vi "Host Approach Retraction2.vi"() -> ()   [LabVIEW 2012]
uses:
  <vilib>/FPGAPlugInAG/PCI-7831R/niLvFpga_Open_PCI-7831R.vi
  <vilib>/rvi/interface/common/dynamic/niFpgaDynamicAddResources.vi
  <vilib>/Utility/error.llb/Error Cluster From Error Code.vi
  <vilib>/rvi/errors/niLvFpgaAdjustHostInterfaceError.vi
  <vilib>/FPGAPlugInAG/Dynamic/niLvFpga_Close_Dynamic.vi
  <vilib>/FPGAPlugInAG/Dynamic/niLvFpga_Run_Dynamic.vi
  <vilib>/rvi/interface/nirviOpenFPGA/nirviOpenFPGA.xnode
  SB130-XPS/Documents/FPGA-project-apporach-retraction/FPGA Bitfiles/Apporach-Retract_FPGATarget2_FPGATargetApproa_XKCjVnL+Gdg.lvbitx
  FPGA Target Approach Retraction2.vi
  <vilib>/rvi/interface/nirviReadWriteControl/nirviReadWriteControl.xnode
  <vilib>/rvi/interface/nirviCloseFPGA/nirviCloseFPGA.xnode
  <vilib>/rvi/interface/nirviMethod/nirviMethod.xnode
  <vilib>/rvi/interface/Simulation/niFpgaSimulationCallBeginRW.vi
  NiFpgaLv.dll
  <vilib>/FPGAPlugInAG/Dynamic/niLvFpga_StartFifo_Dynamic.vi
  <vilib>/rvi/errors/niLvFpgaMergeErrorWithErrorCode.vi
  <vilib>/FPGAPlugInAG/Dynamic/niLvFpga_StopFifo_Dynamic.vi
  <vilib>/FPGAPlugInAG/Dynamic/niLvFpga_ReadFifo_Dynamic.vi
panel:
  in  "Data Acquisition Rate":i32=8000
  out "HV/10":i32[](graph)=[6085, 6084, 6081, 6089, 6083, 6081, 6089, 6086, 6085, 6082, 6090, 6078, 6083, 6081, 6081, 6075, 6082, 6084, 6094, 6094, 6097, 6092, 6083, 6084, 6094, 6085, 6094, 6088, 6085, 6088, 6096, 6079, 6078, 6091, 6099, 6071, 6086, 6086, 6087, 6089, 6086, 6098, 6098, 6101, 6089, 6094, 6083, 6073, 6082, 6086, 6085, 6090, 6084, 6082, 6084, 6084, 6078, 6085, 6094, 6082, 6089, 6088, 6086, 6080, 6087, 6083, 6084, 6082, 6087, 6085, 6079, 6086, 6093, 6085, 6077, 6092, 6081, 6078, 6075, 6072, 6079, 6085, 6084, 6078, 6073, 6090, 6082, 6078, 6088, 6090, 6082, 6098, 6082, 6088, 6079, 6084, 6085, 6084, 6083, 6086]
  out "Tuning Fork":i32[](graph)=[27033, 27029, 27028, 27032, 27032, 27030, 27031, 27032, 27030, 27031, 27034, 27037, 27037, 27035, 27036, 27035, 27030, 27033, 27036, 27034, 27037, 27033, 27030, 27030, 27031, 27025, 27032, 27032, 27032, 27034, 27032, 27032, 27032, 27033, 27029, 27032, 27036, 27032, 27030, 27033, 27031, 27033, 27037, 27036, 27034, 27032, 27032, 27034, 27033, 27032, 27032, 27030, 27029, 27029, 27033, 27033, 27029, 27029, 27033, 27036, 27036, 27033, 27033, 27034, 27033, 27033, 27035, 27033, 27032, 27033, 27032, 27032, 27034, 27036, 27034, 27032, 27035, 27036, 27032, 27036, 27034, 27032, 27032, 27036, 27036, 27033, 27038, 27036, 27033, 27034, 27035, 27032, 27030, 27034, 27039, 27037, 27029, 27033, 27033, 27033]
  in  "Number of Elements":i32=100
  out "Counter Indicator":i32(graph)=-27
  out "Z Indicator":dbl(graph)=30.0
  out "FPGA Output Voltage":dbl(graph)=-0.00824931263923645
  in  "MCL Counter":i64=100
  in  "MCL Divisions":i32=200
  out "MCL Range Indicator":bool=TRUE
  out "Host Counter Indicator":i64=100
  out "Digital Steps per Region":i32=327
  out "Host Counter Output":i32=-27
  in  "Z Position MCL Fine":i32=6000
  out "Host Z Position Indicator":i32=6000
  out "Z Position Range Indicator":bool=TRUE
  out "Z Fine Steps per Region":dbl=0.0049897001602197295
  out "Host Z Output":fxp<+/-,40,30>=29.9384765625
  in  "Manual Approach Start":bool
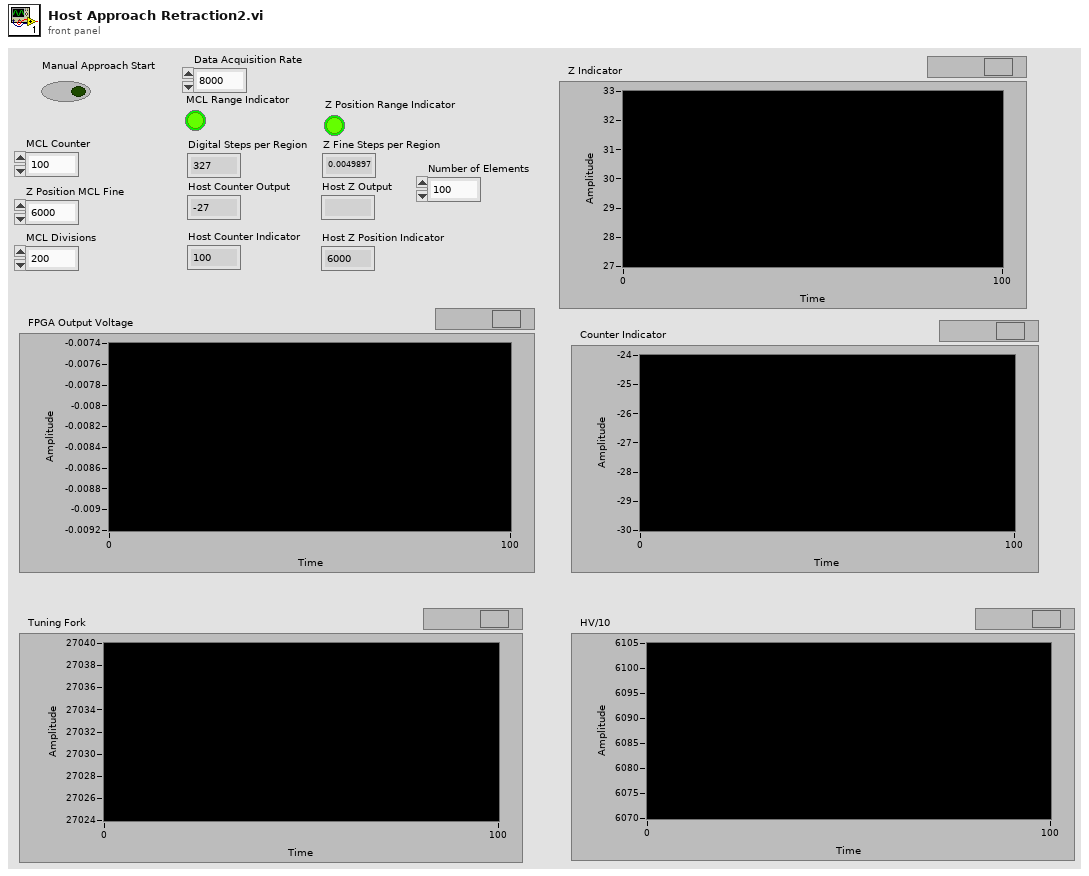
[diagram p1: front panel]
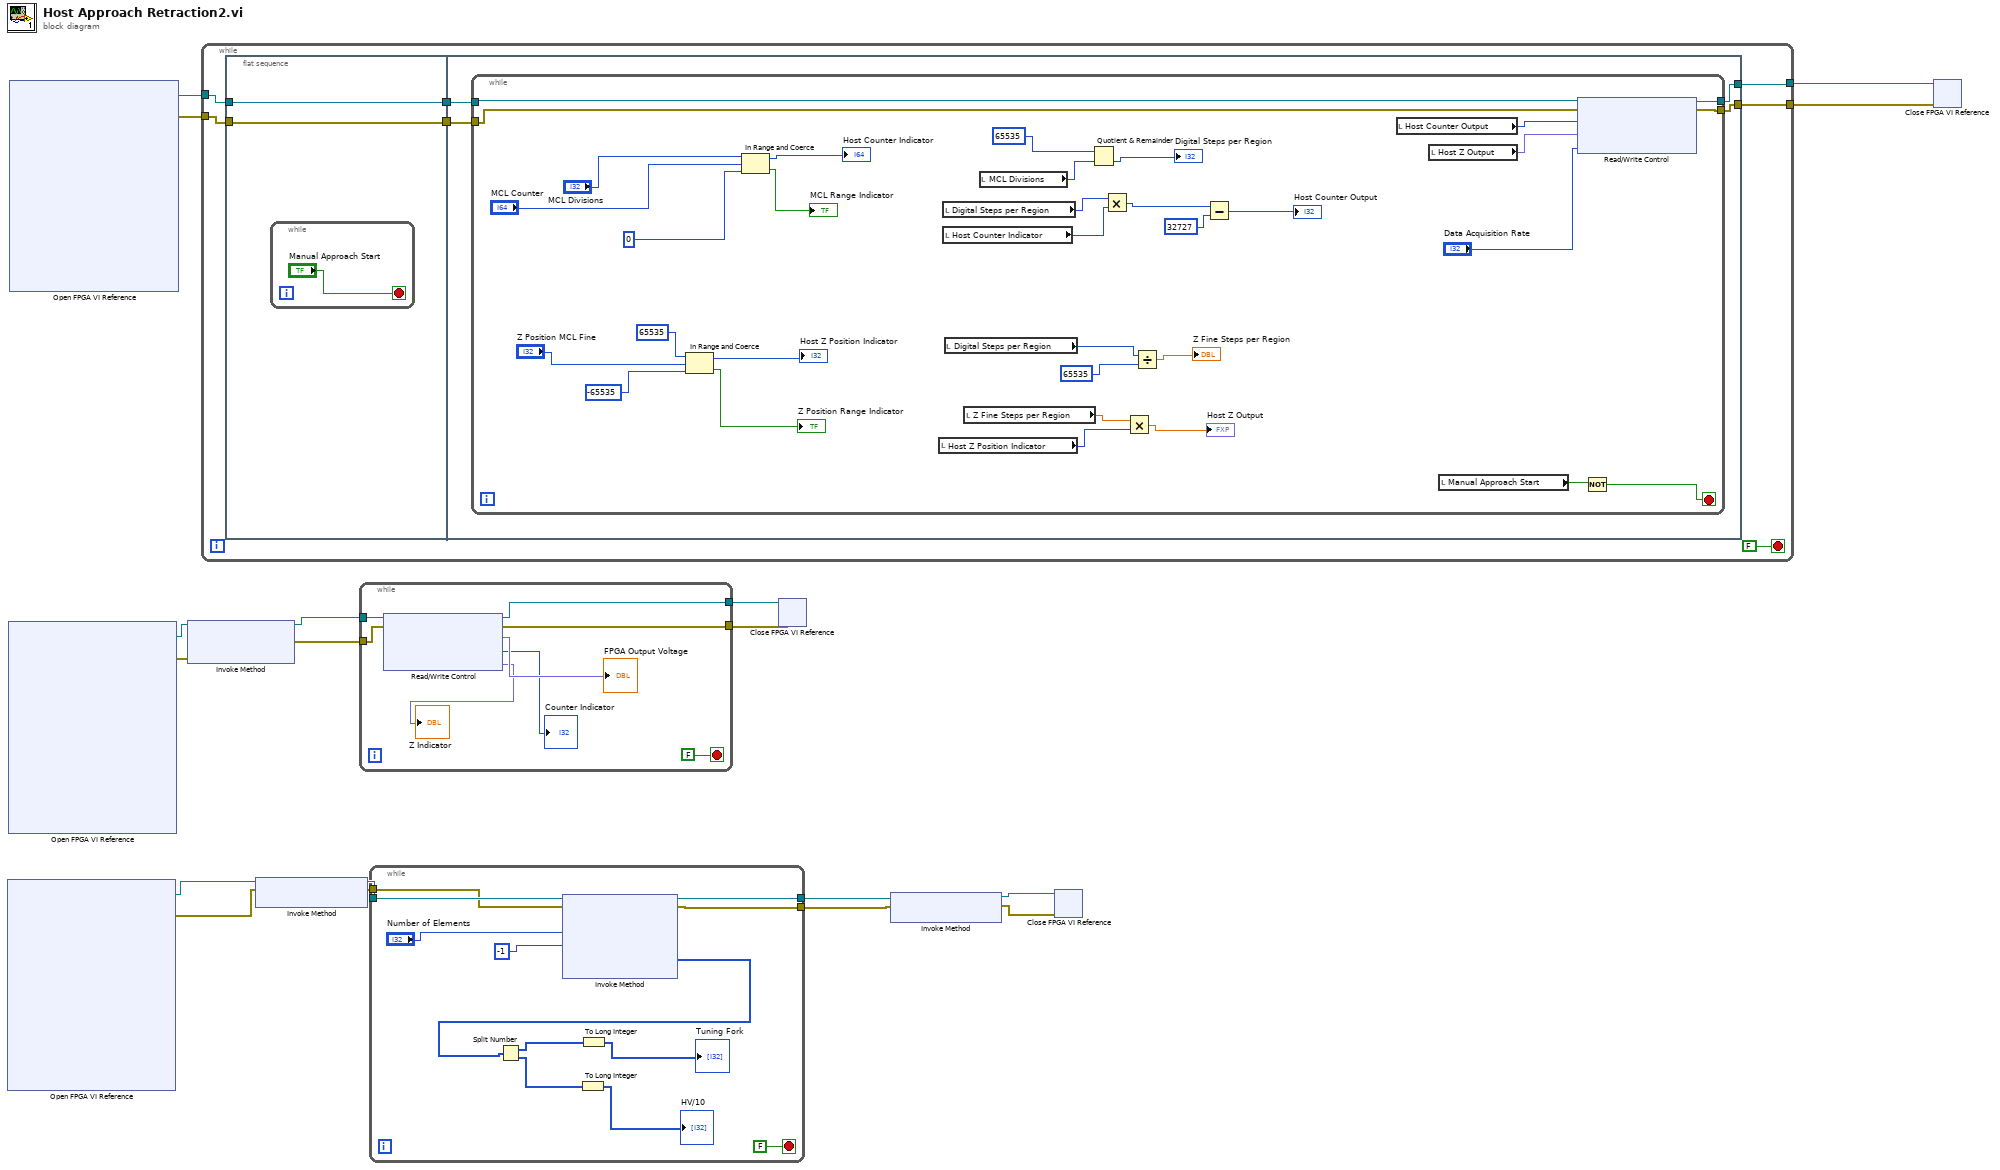
[diagram p0: block diagram]
diagram:
  n1 = xnode "Open FPGA VI Reference"() -> ("FPGA VI Reference Out"=w8:refnum<k20>, "error out"=w7:errorcluster)  [unwired: 2 in]
  n2 = xnode "Open FPGA VI Reference"() -> ("FPGA VI Reference Out"=w10:refnum<k20>, "error out"=w9:errorcluster)  [unwired: 2 in]
  n3 = xnode "Open FPGA VI Reference"() -> ("FPGA VI Reference Out"=w16:refnum<k20>, "error out"=w15:errorcluster)  [unwired: 2 in]
  n4 = xnode "Invoke Method"("FPGA VI Reference In"=w10, "error in"=w9) -> ("FPGA VI Reference Out"=w12:refnum<k20>, "error out"=w11:errorcluster)  [unwired: 1 in]
  n5 = while {
    tunnel: [w24] -> w18
    tunnel: [w23] -> w17
    tunnel: w16 -> [w21]
    tunnel: w15 -> [w19]
    stop <- FALSE stop-if-true
    n6 = flat-sequence {
      tunnel: [w27] -> w22
      tunnel: w21 -> [w27]
      tunnel: [w26] -> w20
      tunnel: w19 -> [w26]
      tunnel: [w30] -> w24
      tunnel: [w29] -> w23
      tunnel: w22 -> [w32]
      tunnel: w20 -> [w31]
      frame #0 {
        n7 = while {
          stop <- "Manual Approach Start" stop-if-true
        }
      }
      frame #1 {
        n8 = while {
          tunnel: w32 -> [w65]
          tunnel: w31 -> [w64]
          tunnel: [w63] -> w30
          tunnel: [w62] -> w29
          stop <- w60 stop-if-true
          n9 = In Range and Coerce(upper limit=65535, x="Z Position MCL Fine", lower limit=-65535) -> (coerced(x)=→"Host Z Position Indicator":i32, In Range?=→"Z Position Range Indicator":bool)
          n10 = In Range and Coerce(upper limit="MCL Divisions", x="MCL Counter", lower limit=0) -> (coerced(x)=→"Host Counter Indicator":i64, In Range?=→"MCL Range Indicator":bool)
          n11 = local read "Host Z Position Indicator"() -> (w36:i32)
          n12 = local read "Digital Steps per Region"() -> (w49:i32)
          n13 = local read "Host Counter Indicator"() -> (w48:i64)
          n14 = local read "Digital Steps per Region"() -> (w40:i32)
          n15 = local read "Z Fine Steps per Region"() -> (w37:dbl)
          n16 = local read "MCL Divisions"() -> (w53:i32)
          n17 = Quotient & Remainder(x=65535, y=w53) -> (floor(x/y)=→"Digital Steps per Region":i32)  [unwired: 1 out]
          n18 = Multiply(x=w49, y=w48) -> (x*y=w50:i64)
          n19 = Multiply(x=w37, y=w36) -> (x*y=→"Host Z Output":dbl)
          n20 = Divide(x=w40, y=65535) -> (x/y=→"Z Fine Steps per Region":dbl)
          n21 = Subtract(x=w50, y=32727) -> (x-y=→"Host Counter Output":i64)
          n22 = local read "Host Counter Output"() -> (w46:i32)
          n23 = local read "Host Z Output"() -> (w34:fxp<+/-,40,30>)
          n24 = local read "Manual Approach Start"() -> (w61:bool)
          n25 = xnode "Read/Write Control"("FPGA VI Reference In"=w65, "error in"=w64, "Counter Output"=w46, "Z Fine Output"=w34, "Data Acquisition Rate"="Data Acquisition Rate") -> ("FPGA VI Reference Out"=w63:refnum<k20>, "error out"=w62:errorcluster)
          n26 = Not(x=w61) -> (.not. x?=w60:bool)
        }
      }
    }
  }
  n27 = xnode "Invoke Method"("FPGA VI Reference In"=w8, "error in"=w7) -> ("FPGA VI Reference Out"=w6:refnum<k20>, "error out"=w5:errorcluster)
  n28 = while {
    tunnel: w12 -> [w72]
    tunnel: w11 -> [w71]
    tunnel: [w70] -> w14
    tunnel: [w69] -> w13
    stop <- FALSE stop-if-true
    n29 = xnode "Read/Write Control"("FPGA VI Reference In"=w72, "error in"=w71) -> ("FPGA VI Reference Out"=w70:refnum<k20>, "error out"=w69:errorcluster, "FPGA Output Voltage"=→"FPGA Output Voltage":fxp<+/-,64,32>, "Counter Indicator"=→"Counter Indicator":i32, "Z Fine Indicator"=→"Z Indicator":fxp<+/-,40,30>)
  }
  n30 = while {
    tunnel: w6 -> [w85]
    tunnel: w5 -> [w84]
    tunnel: [w83] -> w4
    tunnel: [w82] -> w3
    stop <- FALSE stop-if-true
    n31 = xnode "Invoke Method"("FPGA VI Reference In"=w85, "error in"=w84, "Number of Elements"="Number of Elements", "Timeout (ms)"=-1) -> ("FPGA VI Reference Out"=w83:refnum<k20>, "error out"=w82:errorcluster, "Data"=w79:i64[])  [unwired: 1 out]
    n32 = Split Number(x=w79) -> (hi(x)=w78:u32[], lo(x)=w77:u32[])
    n33 = To Long Integer(number=w77) -> (32bit integer=→"HV/10":i32[])
    n34 = To Long Integer(number=w78) -> (32bit integer=→"Tuning Fork":i32[])
  }
  n35 = xnode "Close FPGA VI Reference"("FPGA VI Reference In"=w14, "error in"=w13) -> ()  [unwired: 1 out]
  n36 = xnode "Invoke Method"("FPGA VI Reference In"=w4, "error in"=w3) -> ("FPGA VI Reference Out"=w2:refnum<k20>, "error out"=w1:errorcluster)
  n37 = xnode "Close FPGA VI Reference"("FPGA VI Reference In"=w2, "error in"=w1) -> ()  [unwired: 1 out]
  n38 = xnode "Close FPGA VI Reference"("FPGA VI Reference In"=w18, "error in"=w17) -> ()  [unwired: 1 out]
